vi "Create-client.vi"(8 "error in (no error)":errorcluster, 9 "Module path":path, 10 "Module type":T1=enum."Server", 11 "ModComm in":T2) -> (0 "error out":errorcluster, 3 "ModComm out":T2)   [LabVIEW 2013, in "SLMServer.lvlib" / "SLMServer.lvclass"]
uses:
  SLMServer.lvclass
  Object-reference.ctl
  Supported-module-types.ctl
  Client-connector-diagram.ctl
  UI-messages.ctl
  SLMServer.lvclass/SLMServer.ctl
  Read Server channel.vi
  SA-SLMAPI/Sources/Message.lvclass
panel:
  out "Path":path
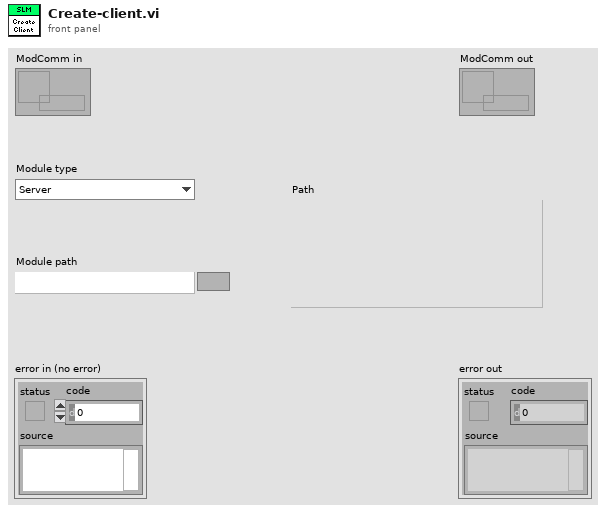
[diagram p1: front panel]
types:
  T1 = typedef "SLMServer.lvlib/SLMServer.lvclass/Supported-module-types.ctl" = enum16{"SLMControl", "PowderDeposition", "CameraVision", "Server", "All", "StrategyParser", "MaterialCharacterization", "StatusMonitor", "SLMSimulation", "LaserCharacterization"}
  T2 = typedef "SLMServer.lvlib/SLMServer.lvclass/Object-reference.ctl" = refnum<data-value>
  T3 = typedef "SLMServer.lvlib/SLMServer.lvclass/UI-messages.ctl" = enum16{"Time out", "User cancel", "Module cancel", "Client inactivity", "Client limit", "Client started"}
  T4 = typedef "SLMServer.lvlib/SLMServer.lvclass/Client-connector-diagram.ctl" = refnum<vi>
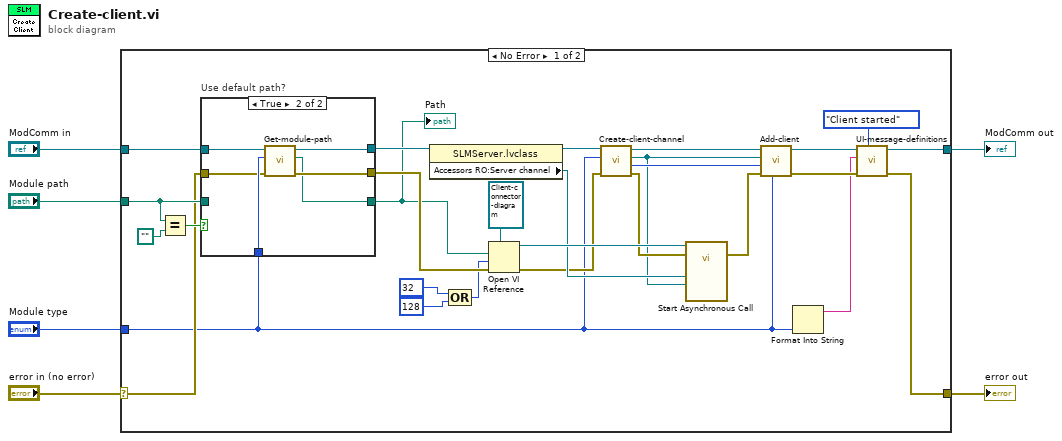
[diagram p0: block diagram]
diagram:
  n1 = case shown="No Error" "error in (no error)" {
    selector: "error in (no error)" -> [w15 w45]
    tunnel: [w13 w45] -> w5
    tunnel: [w8 w44] -> w3
    tunnel: "ModComm in" -> [w34 w44]
    tunnel: "Module path" -> [w31 _]
    tunnel: "Module type" -> [w12 _]
    frame No Error {
      n2 = Equal?(x=w31, y=path "") -> (x = y?=w32:bool)
      n3 = case "Use default path?" shown="True" w32 {
        tunnel: w34 -> [w35 w43]
        tunnel: w12 -> [_ w42]
        tunnel: w15 -> [w36 w41]
        tunnel: [w36 w40] -> w30
        tunnel: [w35 w39] -> w24
        tunnel: [w37 w38] -> w7
        tunnel: w31 -> [w37 _]
        frame False {
        }
        frame True {
          n4 = call "Get-module-path.vi"("error in (no error)"=w41, "Module type"=w42, "ModComm in"=w43) -> ("error out"=w40:errorcluster, "Module path"=w38:path, "ModComm out"=w39:T2)  [unwired: 6 in]
        }
      }
      "Path" <- w7
      n5 = property class="SLMServer.lvclass"(reference=w24) -> (reference out=w22:T2, "Accessors RO:Server channel"=w23:refnum<queue>)  [unwired: 1 in, 1 out]
      n6 = Compound Arithmetic op=OR(32 ("options"), 128 ("options")) -> (w26:i32)
      n7 = Open VI Reference(type specifier VI Refnum (for type only)=T4 refnum, vi path=w7, options=w26, error in (no error)=w30) -> (vi reference=w25:T4, error out=w21:errorcluster)  [unwired: 2 in]
      n8 = call "Create-client-channel.vi"("error in (no error)"=w21, "Client type"=w12, "ModComm in"=w22) -> ("error out"=w20:errorcluster, "Client ID"=w17:i32, "Client channel"=w16:refnum<queue>, "ModComm out"=w19:T2)  [unwired: 5 in]
      n9 = call-by-ref "Start Asynchronous Call"(reference=w25, error in=w20, "Client channel"=w16, "Server channel"=w23) -> (error out=w18:errorcluster)  [unwired: 9 in, 2 out]
      n10 = call "Add-client.vi"("Client type"=w12, "error in (no error)"=w18, "Client ID"=w17, "Client channel"=w16, "ModComm in"=w19) -> ("error out"=w14:errorcluster, "ModComm out"=w9:T2)  [unwired: 5 in]
      n11 = Format Into String(w12) -> (resulting string=w11:string)  [unwired: 3 in, 1 out]
      n12 = call "UI-message-definitions.vi"("Message"=UI-messages."Client started", "error in (no error)"=w14, "Additional text"=w11, "ModComm in"=w9) -> ("error out"=w13:errorcluster, "ModComm out"=w8:T2)  [unwired: 6 in]
    }
    frame Error {
    }
  }
  "error out" <- w5
  "ModComm out" <- w3
